vi "InitUserTable.vi"(8 "Error in":errorcluster caption="Error in (no error)", 11 "User Table":refnum<vi>) -> (0 "error out":errorcluster)   [LabVIEW 2020, in "Login-UI.lvlib"]
uses:
  Login-UI.lvlib
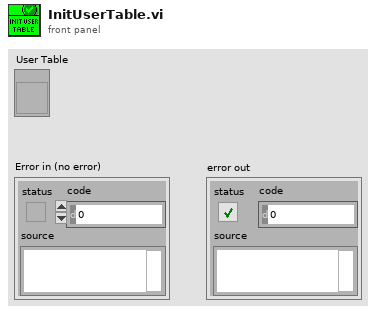
[diagram p1: front panel]
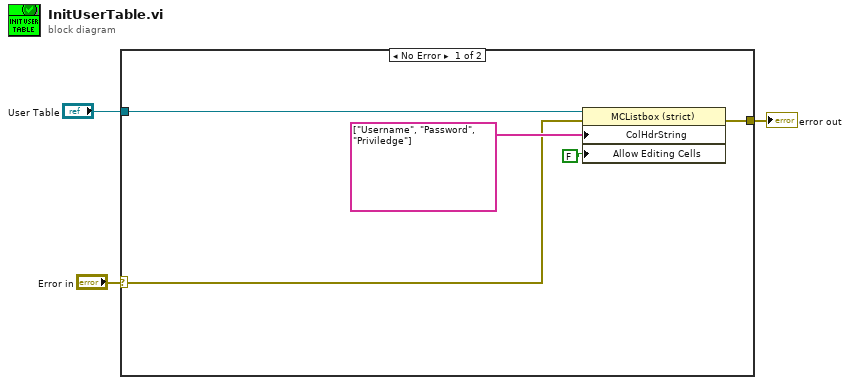
[diagram p0: block diagram]
diagram:
  n1 = case shown="No Error" "Error in" {
    selector: "Error in" -> [w4 w9]
    tunnel: "User Table" -> [w8 _]
    tunnel: [w6 w9] -> w1
    frame No Error {
      n2 = property class="MCListbox (strict)"(reference=w8, error in=w4, "ColHdrString"=string[] ["Username", "Password", "Priviledge"] ("Column Header Strings[]"), "Allow Editing Cells"=FALSE) -> (error out=w6:errorcluster)  [unwired: 1 out]
    }
    frame Error {
    }
  }
  "error out" <- w1
